vi "例程43-生成二维数组.vi"() -> ()   [LabVIEW 2016]
panel:
  out "数组":dbl[][](array[numeric])
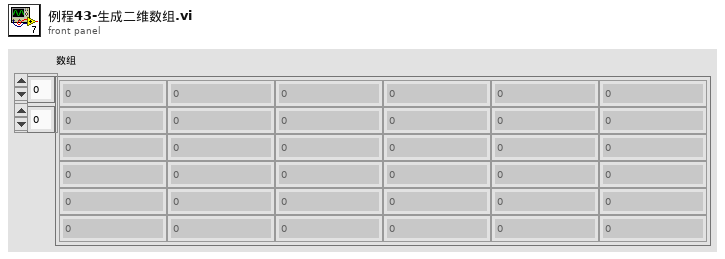
[diagram p1: front panel]
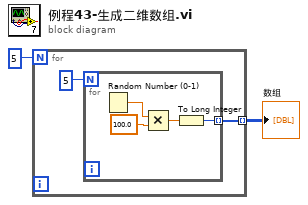
[diagram p0: block diagram]
diagram:
  n1 = for {
    N: 5 -> [_]
    tunnel: [w3] -> w1 mode=indexing
    n2 = for {
      N: 5 -> [_]
      tunnel: [w5] -> w3 mode=indexing
      n3 = Random Number (0-1)() -> (number: 0 to 1=w7:dbl)
      n4 = Multiply(x=w7, y=100.0) -> (x*y=w6:dbl)
      n5 = To Long Integer(number=w6) -> (32bit integer=w5:i32)
    }
  }
  "数组" <- w1
